vi "Cumulative Sum.vi"(8 "error in (no error)":errorcluster, 11 "Value In":i32) -> (0 "error out":errorcluster, 3 "Cumulative Sum":i32)   [LabVIEW 2023]
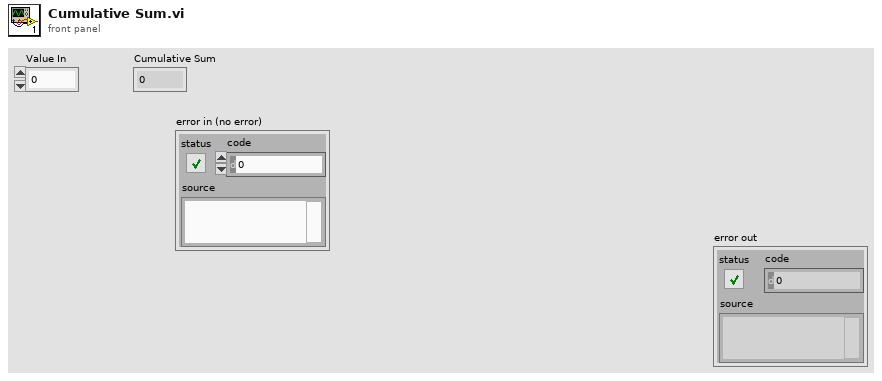
[diagram p1: front panel]
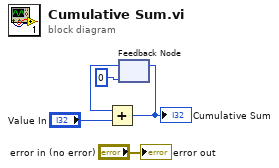
[diagram p0: block diagram]
diagram:
  n1 = feedback #1(0) -> (w2:i32)
  n2 = Add(x=w2, y="Value In") -> (x+y=w3:i32)
  "Cumulative Sum" <- w3
  n3 = feedback-in #1(w3) -> ()
  "error out" <- "error in (no error)"
